vi "DB Tools Create Table.vi"(4 "use file? (F)":bool, 5 "primary key (-1)":i32=-1, 6 "error in (no error)":errorcluster, 7 "column information":T1[](array[typedef]), 8 "table":string, 9 "connection reference":T3) -> (0 "error out":errorcluster, 3 "connection reference out":T3)   [LabVIEW 2013, in "NI_Database_API_64.lvlib"]
doc: "Creates a new table in the database identified by <B>connection reference</B>. The <B>table</B> and <B>column information</B> inputs describe the name of the table and the properties of each column in the table, respectively."
uses:
  NI_Database_API_64.lvlib
  Connection.llb/Conn ObjectReference.ctl
  DB Tools Column Info.ctl
  DB Tools DataTypes.ctl
  Connection.llb/Conn Execute.vi
  Recordset.llb/Rec Destroy - Connection.vi
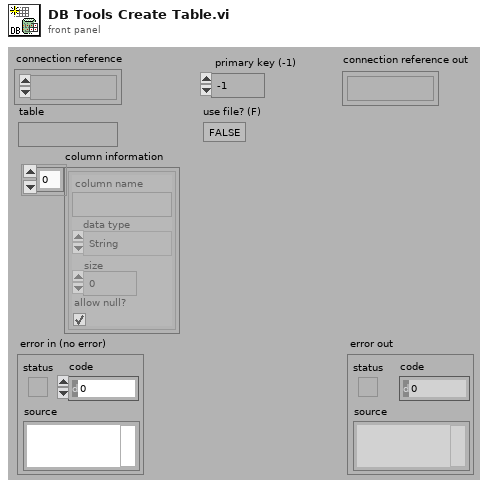
[diagram p1: front panel]
types:
  T1 = typedef "NI_Database_API_64.lvlib/DB Tools Column Info.ctl" = cluster{"column name":string, "data type":T2, "size":i32, "allow null?":bool}
  T2 = typedef "NI_Database_API_64.lvlib/DB Tools DataTypes.ctl" = enum16{"String", "Long (I32)", "Single (SGL)", "Double (DBL)", "Date/Time", "Binary"}
  T3 = typedef "NI_Database_API_64.lvlib/Conn ObjectReference.ctl" = refnum<k1>
  T4 = typedef "NI_Database_API_64.lvlib/DB Tools Database.ctl" = enum16{"dBase", "Jet", "SQL Server", "Oracle"}
  T5 = typedef "NI_Database_API_64.lvlib/Rec ObjectReference.ctl" = refnum<k1>
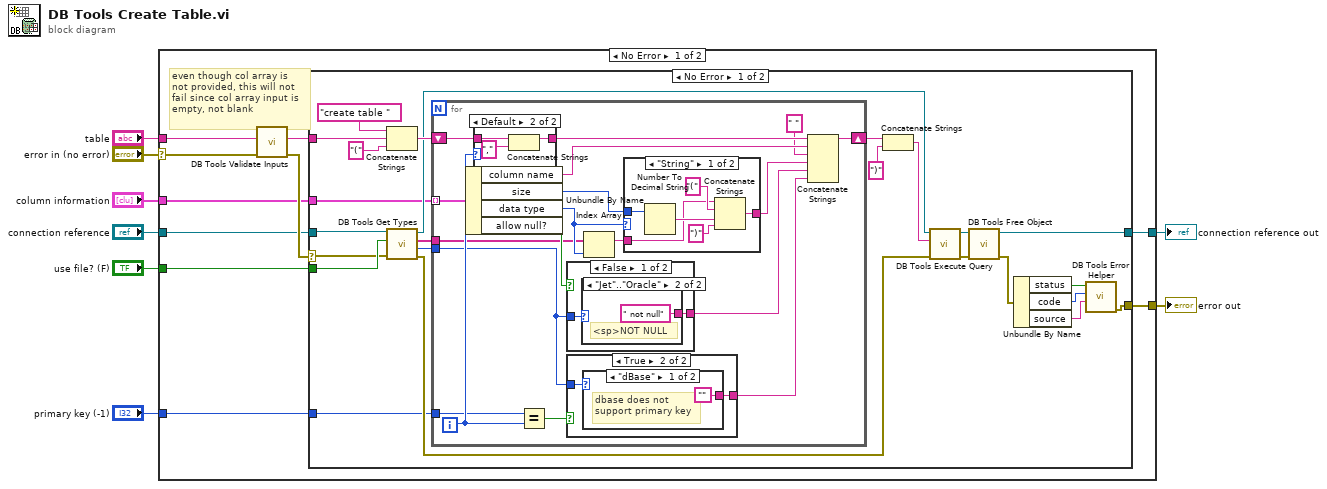
[diagram p0: block diagram]
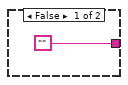
[diagram p2: hidden frame]
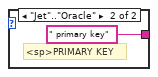
[diagram p3: hidden frame]
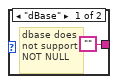
[diagram p4: hidden frame]
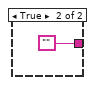
[diagram p5: hidden frame]
diagram:
  n1 = case shown="No Error" "error in (no error)" {
    selector: "error in (no error)" -> [w9 w85]
    tunnel: "table" -> [w18 _]
    tunnel: [w15 w85] -> w7
    tunnel: "connection reference" -> [w14 w84]
    tunnel: [w13 w84] -> w5
    tunnel: "primary key (-1)" -> [w12 _]
    tunnel: "column information" -> [w11 _]
    tunnel: "use file? (F)" -> [w10 _]
    frame No Error {
      # "even though col array is \nnot provided, this will not \nfail since col array input is \nempty, not blank"
      n2 = call "DB Tools Validate Inputs.vi"("error in (no error)"=w9, "table"=w18) -> ("error out"=w17:errorcluster, "table out"=w16:string)  [unwired: 3 in, 1 out]
      n3 = case shown="No Error" w17 {
        selector: w17 -> [w19 w83]
        tunnel: w16 -> [w40 _]
        tunnel: w14 -> [w20 w82]
        tunnel: [w33 w82] -> w13
        tunnel: [w24 w83] -> w15
        tunnel: w12 -> [w23 _]
        tunnel: w11 -> [w21 _]
        tunnel: w10 -> [w22 _]
        frame No Error {
          n4 = Concatenate Strings("create table " ("Substring"), w40, "(" ("Substring")) -> (w39:string)
          n5 = call "DB Tools Get Types.vi"("error in (no error)"=w19, "file?"=w22, "connection reference"=w20) -> ("error out"=w30:errorcluster, "database"=w29:T4, "data types"=w31:string[], "connection reference out"=w36:T3)  [unwired: 1 in]
          n6 = for {
            tunnel: w21 -> [w60] mode=indexing
            shift-right: [w54] -> w38
            shift-left: w39 -> [w59]
            tunnel: w31 -> [w49]
            tunnel: w29 -> [w44]
            tunnel: w23 -> [w43]
            i -> [w57]
            n7 = Unbundle By Name(w60) -> ("column name"=w52:string, "size"=w47:i32, "data type"=w50:T2, "allow null?"=w58:bool)
            n8 = case shown="Default" w57 {
              tunnel: [w78 w81] -> w53
              tunnel: w59 -> [w78 w79]
              frame 0 {
              }
              frame Default {
                n9 = Concatenate Strings(w79, "," ("Substring")) -> (w81:string)
              }
            }
            n10 = Equal?(x=w43, y=w57) -> (x = y?=w56:bool)
            n11 = case shown="False" w58 {
              tunnel: w44 -> [w67 _]
              tunnel: [w66 ""] -> w46
              frame False {
                n12 = case shown="\"Jet\"..\"Oracle\"" w67 {
                  tunnel: ["" " not null"] -> w66
                  frame "dBase" {
                    # "dbase does\nnot support\nNOT NULL"
                  }
                  frame "Jet".."Oracle" {
                    # "<sp>NOT NULL"
                  }
                }
              }
              frame True {
              }
            }
            n13 = case shown="True" w56 {
              tunnel: ["" w63] -> w45
              tunnel: w44 -> [_ w62]
              frame False {
              }
              frame True {
                n14 = case shown="\"dBase\"" w62 {
                  tunnel: ["" " primary key"] -> w63
                  frame "dBase" {
                    # "dbase does not \nsupport primary key"
                  }
                  frame "Jet".."Oracle" {
                    # "<sp>PRIMARY KEY"
                  }
                }
              }
            }
            n15 = Index Array(array=w49, index=w50) -> (element=w48:string)
            n16 = case shown="\"String\"" w50 {
              tunnel: w48 -> [w71 w77]
              tunnel: [w73 w77] -> w55
              tunnel: w47 -> [w72 _]
              frame "String" {
                n17 = Number To Decimal String(number=w72) -> (decimal integer string=w75:string)  [unwired: 1 in]
                n18 = Concatenate Strings(w71, "(" ("Substring"), w75, ")" ("Substring")) -> (w73:string)
              }
              frame "Long (I32)".."Binary" {
              }
            }
            n19 = Concatenate Strings(w53, w52, " " ("Substring"), w55, w46, w45) -> (w54:string)
          }
          n20 = Concatenate Strings(w38, ")" ("Substring")) -> (w32:string)
          n21 = call-poly "DB Tools Execute Query.vi"("error in (no error)"=w30, "SQL query"=w32, "connection reference"=w36) -> ("error out"=w35:errorcluster, "recordset reference"=w34:T5)  [unwired: 5 in]
          n22 = call-poly "DB Tools Free Object.vi"("error in (no error)"=w35, "recordset reference"=w34) -> ("error out"=w25:errorcluster, "connection reference"=w33:T3)  [unwired: 8 in]
          n23 = Unbundle By Name(w25) -> ("status"=w27:bool, "code"=w28:i32, "source"=w26:string)
          n24 = call "DB Tools Error Helper.vi"("source"=w26, "code"=w28, "status"=w27) -> ("error out"=w24:errorcluster)  [unwired: 8 in]
        }
        frame Error {
        }
      }
    }
    frame Error {
    }
  }
  "error out" <- w7
  "connection reference out" <- w5
